vi "TRAFFIC Project.vi"() -> ()   [LabVIEW 2018]
panel:
  in  "?":bool
  in  "Stop":bool
  in  "Clock delay in ms":u32
  out "Red":bool
  out "Yellow":bool
  out "Green":bool
  out "g 2":bool
  out "f 2":bool
  out "e 2":bool
  out "d 2":bool
  out "c 2":bool
  out "b 2":bool
  out "a 2":bool
  out "g":bool
  out "f":bool
  out "e":bool
  out "d":bool
  out "c":bool
  out "b":bool
  out "a":bool
  out "B 8":bool
  out "B 7":bool
  out "B 6":bool
  out "B 5":bool
  out "B 4":bool
  out "B 3":bool
  out "B 2":bool
  out "B1":bool
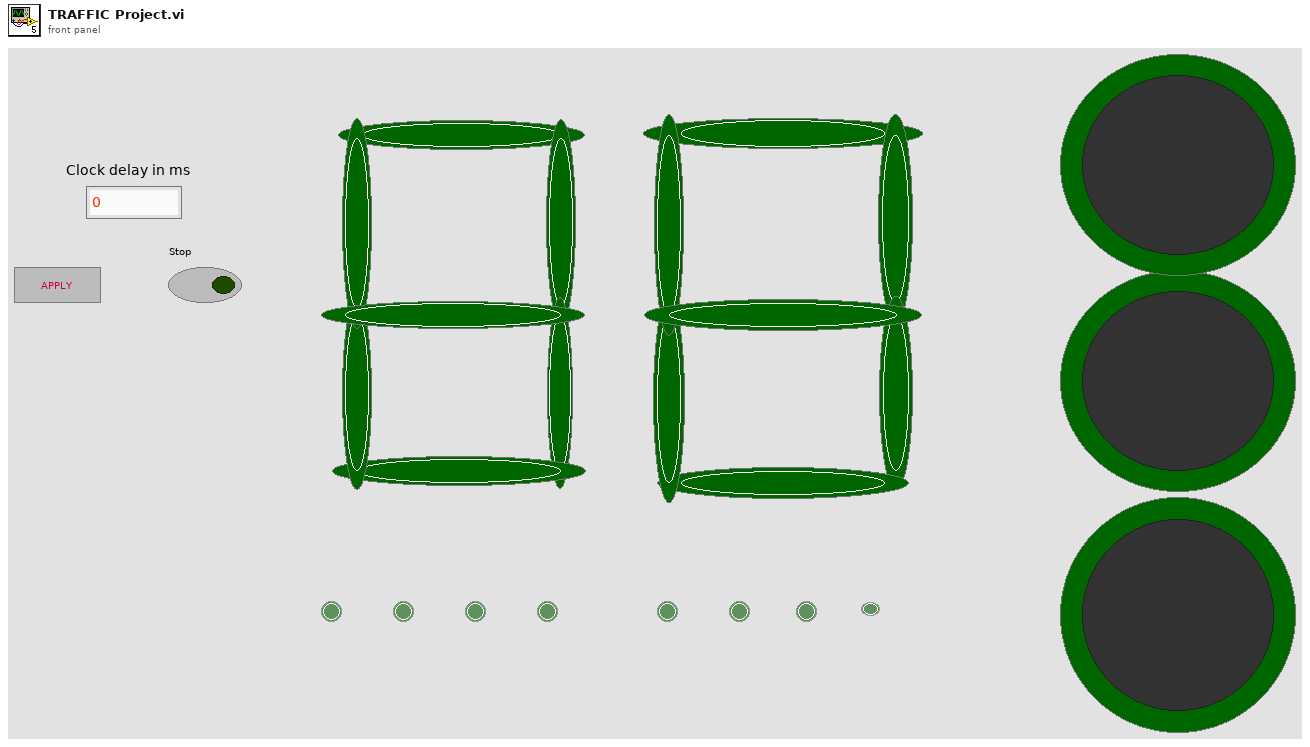
[diagram p1: front panel]
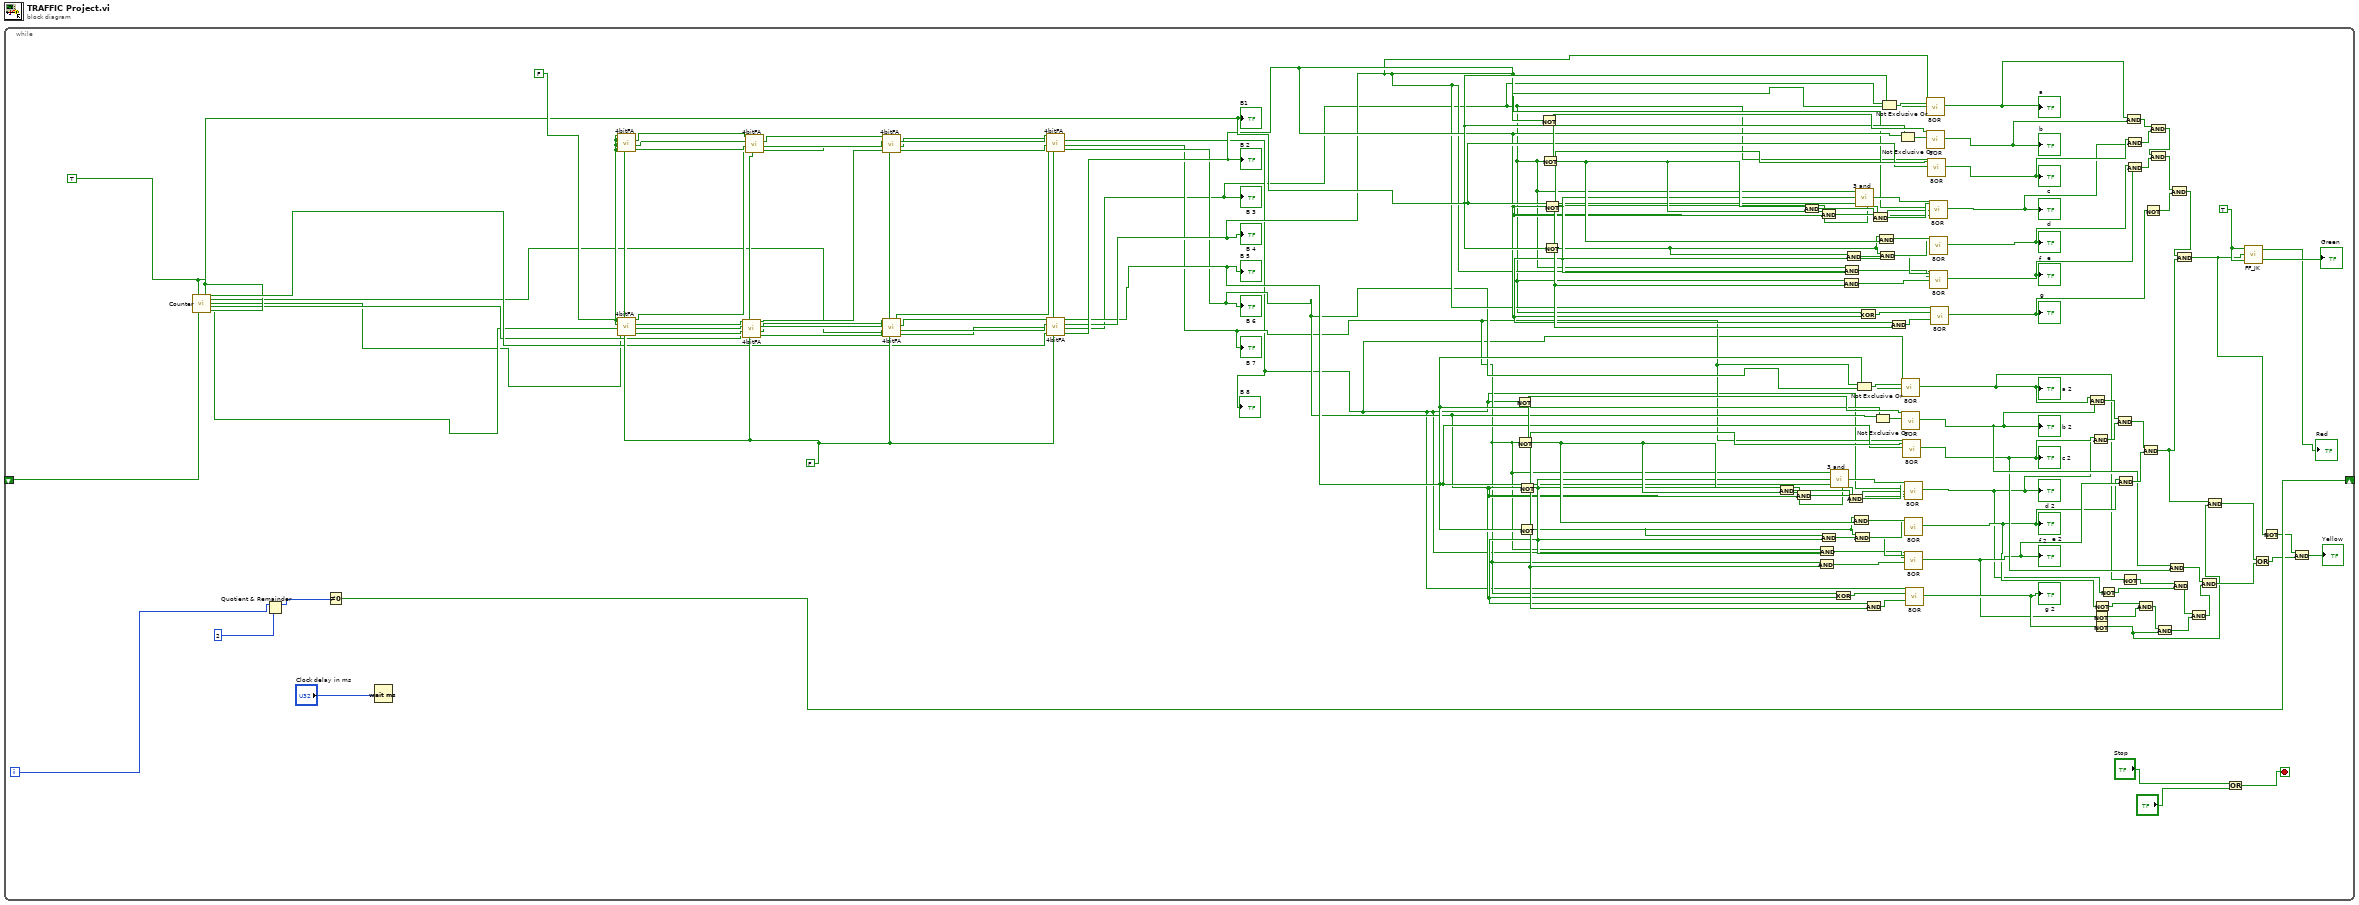
[diagram p0: block diagram]
diagram:
  n1 = while {
    shift-right: [w62] -> _
    shift-left: _ -> [w63]
    i -> [w66]
    stop <- w1 stop-if-true
    w31 = TRUE
    w67 = TRUE
    w101 = FALSE
    w123 = FALSE
    n2 = call "Counter.vi"("T0"=w67, "T4"=w67, "T1"=w67, "T2"=w67, "T3"=w67, "clock"=w63, "T5"=w67) -> ("A0"=w57:bool, "A1"=w68:bool, "A2"=w61:bool, "A4"=w58:bool, "A3"=w60:bool, "A5\nA5"=w59:bool)  [unwired: 3 in]
    "B1" <- w57
    n3 = Quotient & Remainder(x=w66, y=2) -> (x-y*floor(x/y)=w64:i32)  [unwired: 1 out]
    n4 = Not Equal To 0?(x=w64) -> (x != 0?=w62:bool)
    n5 = Wait (ms)(milliseconds to wait="Clock delay in ms") -> ()  [unwired: 1 out]
    n6 = call "4bitFA.vi"("Cin"=w123, "A1"=w58, "A2"=w59, "A4"=w101, "A8"=w101) -> ("B2"=w120:bool, "B4"=w121:bool, "B8"=w122:bool, "B1"=w104:bool, "Cout"=w127:bool)
    n7 = call "4bitFA.vi"("Cin"=w127, "A1"=w101, "A2"=w101, "A4"=w101, "A8"=w101) -> ("B2"=w111:bool, "B4"=w112:bool, "B8"=w113:bool)  [unwired: 2 out]
    n8 = call "4bitFA.vi"("Cin"=w123, "A1"=w60, "A2"=w120, "A4"=w121, "A8"=w122) -> ("B2"=w117:bool, "B4"=w118:bool, "B8"=w119:bool, "B1"=w103:bool, "Cout"=w126:bool)
    n9 = call "4bitFA.vi"("Cin"=w126, "A1"=w104, "A2"=w111, "A4"=w112, "A8"=w113) -> ("B2"=w108:bool, "B4"=w109:bool, "B8"=w110:bool)  [unwired: 2 out]
    n10 = call "4bitFA.vi"("Cin"=w123, "A1"=w61, "A2"=w117, "A4"=w118, "A8"=w119) -> ("B2"=w114:bool, "B4"=w115:bool, "B8"=w116:bool, "B1"=w102:bool, "Cout"=w125:bool)
    n11 = call "4bitFA.vi"("Cin"=w125, "A1"=w103, "A2"=w108, "A4"=w109, "A8"=w110) -> ("B2"=w105:bool, "B4"=w106:bool, "B8"=w107:bool)  [unwired: 2 out]
    n12 = call "4bitFA.vi"("Cin"=w123, "A1"=w68, "A2"=w114, "A4"=w115, "A8"=w116) -> ("B2"=w56:bool, "B4"=w50:bool, "B8"=w55:bool, "B1"=w54:bool, "Cout"=w124:bool)
    "B 2" <- w56
    "B 3" <- w50
    "B 4" <- w55
    "B 5" <- w54
    n13 = call "4bitFA.vi"("Cin"=w124, "A1"=w102, "A2"=w105, "A4"=w106, "A8"=w107) -> ("B2"=w53:bool, "B4"=w52:bool, "B8"=w51:bool)  [unwired: 2 out]
    "B 6" <- w53
    "B 7" <- w52
    "B 8" <- w51
    n14 = Not(x=w51) -> ()  [unwired: 1 out]
    n15 = Not(x=w52) -> (.not. x?=w77:bool)
    n16 = Not(x=w54) -> (.not. x?=w71:bool)
    n17 = Not(x=w53) -> (.not. x?=w73:bool)
    n18 = Not(x=w55) -> ()  [unwired: 1 out]
    n19 = Not(x=w50) -> (.not. x?=w93:bool)
    n20 = Not(x=w57) -> (.not. x?=w87:bool)
    n21 = Not(x=w56) -> (.not. x?=w89:bool)
    n22 = And(x=w77, y=w53) -> (x .and. y?=w79:bool)
    n23 = And(x=w77, y=w71) -> (x .and. y?=w80:bool)
    n24 = And(x=w93, y=w56) -> (x .and. y?=w95:bool)
    n25 = And(x=w52, y=w71) -> (x .and. y?=w72:bool)
    n26 = And(x=w52, y=w73) -> (x .and. y?=w74:bool)
    n27 = And(x=w93, y=w87) -> (x .and. y?=w96:bool)
    n28 = And(x=w71, y=w73) -> (x .and. y?=w75:bool)
    n29 = call "3 and.vi"("Boolean 3"=w54, "Boolean 2"=w73, "Boolean"=w52) -> ("Boolean 4"=w82:bool)
    n30 = Exclusive Or(1:w53, 2:w52) -> (0:w69:bool)
    n31 = And(x=w50, y=w87) -> (x .and. y?=w88:bool)
    n32 = And(x=w50, y=w89) -> (x .and. y?=w90:bool)
    n33 = And(x=w87, y=w89) -> (x .and. y?=w91:bool)
    n34 = And(x=w53, y=w71) -> (x .and. y?=w81:bool)
    n35 = And(x=w71, y=w77) -> (x .and. y?=w78:bool)
    n36 = And(x=w71, y=w53) -> (x .and. y?=w76:bool)
    n37 = call "3 and.vi"("Boolean 3"=w57, "Boolean 2"=w89, "Boolean"=w50) -> ("Boolean 4"=w98:bool)
    n38 = Not Exclusive Or(1:w54, 2:w52) -> (0:w84:bool)
    n39 = Exclusive Or(1:w56, 2:w50) -> (0:w85:bool)
    n40 = And(x=w53, y=w71) -> (x .and. y?=w70:bool)
    n41 = And(x=w56, y=w87) -> (x .and. y?=w97:bool)
    n42 = Not Exclusive Or(1:w54, 2:w53) -> (0:w83:bool)
    n43 = And(x=w87, y=w93) -> (x .and. y?=w94:bool)
    n44 = And(x=w87, y=w56) -> (x .and. y?=w92:bool)
    n45 = Not Exclusive Or(1:w57, 2:w50) -> (0:w100:bool)
    n46 = And(x=w56, y=w87) -> (x .and. y?=w86:bool)
    n47 = Not Exclusive Or(1:w57, 2:w56) -> (0:w99:bool)
    n48 = call "8OR.vi"("Boolean"=w51, "Boolean 2"=w53, "Boolean 3"=w84) -> ("Boolean 9"=w19:bool)  [unwired: 24 in]
    "a 2" <- w19
    n49 = call "8OR.vi"("Boolean"=w77, "Boolean 3"=w83) -> ("Boolean 9"=w30:bool)  [unwired: 25 in]
    "b 2" <- w30
    n50 = call "8OR.vi"("Boolean"=w52, "Boolean 2"=w73, "Boolean 4"=w54) -> ("Boolean 9"=w29:bool)  [unwired: 24 in]
    "c 2" <- w29
    n51 = call "8OR.vi"("Boolean"=w82, "Boolean 2"=w81, "Boolean 5"=w80, "Boolean 6"=w51, "Boolean 7"=w79) -> ("Boolean 9"=w20:bool)  [unwired: 22 in]
    "d 2" <- w20
    n52 = call "8OR.vi"("Boolean"=w78, "Boolean 2"=w76) -> ("Boolean 9"=w21:bool)  [unwired: 25 in]
    "e 2" <- w21
    n53 = call "8OR.vi"("Boolean"=w51, "Boolean 2"=w75, "Boolean 3"=w74, "Boolean 5"=w72) -> ("Boolean 9"=w22:bool)  [unwired: 23 in]
    "f 2" <- w22
    n54 = call "8OR.vi"("Boolean"=w51, "Boolean 3"=w69, "Boolean 6"=w70) -> ("Boolean 9"=w23:bool)  [unwired: 24 in]
    "g 2" <- w23
    n55 = call "8OR.vi"("Boolean"=w55, "Boolean 2"=w56, "Boolean 3"=w100) -> ("Boolean 9"=w49:bool)  [unwired: 24 in]
    "a" <- w49
    n56 = call "8OR.vi"("Boolean"=w93, "Boolean 3"=w99) -> ("Boolean 9"=w48:bool)  [unwired: 25 in]
    "b" <- w48
    n57 = call "8OR.vi"("Boolean"=w50, "Boolean 2"=w89, "Boolean 4"=w57) -> ("Boolean 9"=w47:bool)  [unwired: 24 in]
    "c" <- w47
    n58 = call "8OR.vi"("Boolean"=w98, "Boolean 2"=w97, "Boolean 5"=w96, "Boolean 6"=w55, "Boolean 7"=w95) -> ("Boolean 9"=w46:bool)  [unwired: 22 in]
    "d" <- w46
    n59 = call "8OR.vi"("Boolean"=w94, "Boolean 2"=w92) -> ("Boolean 9"=w45:bool)  [unwired: 25 in]
    "e" <- w45
    n60 = call "8OR.vi"("Boolean"=w55, "Boolean 2"=w91, "Boolean 3"=w90, "Boolean 5"=w88) -> ("Boolean 9"=w44:bool)  [unwired: 23 in]
    "f" <- w44
    n61 = call "8OR.vi"("Boolean"=w55, "Boolean 3"=w85, "Boolean 6"=w86) -> ("Boolean 9"=w33:bool)  [unwired: 24 in]
    "g" <- w33
    n62 = And(x=w19, y=w30) -> (x .and. y?=w37:bool)
    n63 = And(x=w29, y=w20) -> (x .and. y?=w38:bool)
    n64 = Not(x=w22) -> (.not. x?=w25:bool)
    n65 = Not(x=w23) -> (.not. x?=w12:bool)
    n66 = Not(x=w21) -> (.not. x?=w26:bool)
    n67 = Not(x=w20) -> (.not. x?=w27:bool)
    n68 = And(x=w37, y=w38) -> (x .and. y?=w36:bool)
    n69 = And(x=w21, y=w22) -> (x .and. y?=w39:bool)
    n70 = Not(x=w19) -> (.not. x?=w28:bool)
    n71 = And(x=w49, y=w48) -> (x .and. y?=w43:bool)
    n72 = And(x=w47, y=w46) -> (x .and. y?=w42:bool)
    n73 = And(x=w45, y=w44) -> (x .and. y?=w41:bool)
    n74 = And(x=w26, y=w25) -> (x .and. y?=w24:bool)
    n75 = And(x=w36, y=w39) -> (x .and. y?=w13:bool)
    n76 = Not(x=w33) -> (.not. x?=w32:bool)
    n77 = And(x=w43, y=w42) -> (x .and. y?=w40:bool)
    n78 = And(x=w40, y=w41) -> (x .and. y?=w35:bool)
    n79 = And(x=w24, y=w12) -> (x .and. y?=w18:bool)
    n80 = And(x=w30, y=w29) -> (x .and. y?=w16:bool)
    n81 = And(x=w35, y=w32) -> (x .and. y?=w34:bool)
    n82 = And(x=w28, y=w27) -> (x .and. y?=w17:bool)
    n83 = And(x=w34, y=w13) -> (x .and. y?=w7:bool)
    n84 = And(x=w17, y=w18) -> (x .and. y?=w15:bool)
    n85 = And(x=w16, y=w15) -> (x .and. y?=w14:bool)
    n86 = And(x=w13, y=w12) -> (x .and. y?=w11:bool)
    n87 = Or(x="Stop", y="?") -> (x .or. y?=w1:bool)
    n88 = call "FF_JK.vi"("K"=w31, "Clock"=w7, "J"=w31) -> ("Q!"=→"Green":bool, "Q"=→"Red":bool)
    n89 = Or(x=w11, y=w14) -> (x .or. y?=w5:bool)
    n90 = Not(x=w7) -> (.not. x?=w6:bool)
    n91 = And(x=w6, y=w5) -> (x .and. y?=→"Yellow":bool)
  }
